vi "Chart_Data_Packer.vi"(0 "DataCluster":T2={"Core"={"Current VI Reference"=refnum, "Close Panel on Exit?"=FALSE, "Exit"=FALSE, "Initialized?"=FALSE}, "Connections"={"cDAQ"={"Task"="", "Connected"=FALSE, "Active"=FALSE, "ID"=""}, "Camera"={"Session"="", "Connected"=FALSE, "Active"=FALSE, "Placeholder"=refnum}, "PSU"={"Port"="", "Connected"=FALSE, "Active"=FALSE}, "Arduino"={"Port"="", "Connected"=FALSE, "Active"=FALSE}}, "Data Acquisition"={"Setup"={"Label"="", "Operator"="", "Notes"="", "TempGrad"=1.0, "TargetTemp"=1.0, "Sample Volume"=1.0}, "Camera"={"Image"=refnum, "Save Image"=refnum, "Image Frequency"=20, "Rectangle"={"Left"=0, "Top"=0, "Right"=0, "Bottom"=0, "Rotation"=0.0}, "Calibration"={"Top Left"={"X"=0.0, "Y"=0.0}, "Top Right"={"X"=0.0, "Y"=0.0}, "Bottom Left"={"X"=0.0, "Y"=0.0}, "Bottom Right"={"X"=0.0, "Y"=0.0}, "Fixpoint"={"X"=0.0, "Y"=0.0}, "Scan Area"=0.0, "Fixpoint Area"=0.0, "Well Pixels"=[], "Valid"=FALSE}, "FocusPos"=0, "Display Mapping"=10, "Camera Mode"=10}, "Thermistor"={"Sample Size"=1, "Calibration"={"B0.100"=[], "R25"=[], "c"=[], "State"=[], "V_S"=5.0, "R_S"=100.0}, "Timing Mode"=14713}, "Partition"={"Data"=[], "Cell Label"="", "Cell Color"=0, "Height"=10, "Width"=16, "Grid"=[]}, "Queue"={"Size"=1, "Queue"=refnum}, "Sample Rate"=1, "Active"=FALSE, "Ready"=FALSE, "Graph Mode"=0, "Gradient Buffer"=2}, "Control"={"Sample Rate"=1, "PID gains"={"proportional gain (Kc)"=1.0, "integral time (Ti, min)"=0.01, "derivative time (Td, min)"=0.0}}, "Manual Temp Control"={"TargetTemp"=1.0, "Mode"=0, "Active"=FALSE}} {"Manual Temp Control"."Mode" items=["Cool", "Heat"]; "Manual Temp Control"."TargetTemp" min=-40.0 max=40.0 step=0.5 format="%#_g °C"; "Control"."PID gains"."derivative time (Td, min)" format="%.3f"; "Control"."PID gains"."integral time (Ti, min)" format="%.3f"; "Control"."PID gains"."proportional gain (Kc)" format="%.3f"; "Control"."Sample Rate" min=1 max=20 step=1 format="%.0f Samples/sec"; "Data Acquisition"."Gradient Buffer" min=2 max=30 step=1; "Data Acquisition"."Graph Mode" items=["Thermistor Temperature", "Camera Temperature"]; "Data Acquisition"."Thermistor"."Timing Mode" items=["Automatic"=16097, "High Resolution"=10195, "High Speed"=14712, "Best 50 Hz Rejection"=14713, "Best 60 Hz Rejection"=14714, "Custom"=10137]; "Data Acquisition"."Thermistor"."Calibration"."R_S" min=0.1 max=1000.0 format="%#_g kOhm"; "Data Acquisition"."Thermistor"."Calibration"."V_S" min=5.0 max=48.0 format="%#_g V"; "Data Acquisition"."Thermistor"."Calibration"."R25" min=0.1 max=1000.0 format="%#_g kOhm"; "Data Acquisition"."Thermistor"."Calibration"."B0.100" min=100.0 max=10000.0 format="%#_g K"; "Data Acquisition"."Thermistor"."Sample Size" min=1 max=200; "Data Acquisition"."Sample Rate" min=20 max=240 format="%.0f samples/min"; "Data Acquisition"."Queue"."Size" min=1 max=200; "Data Acquisition"."Camera"."Camera Mode" items=["Temperature Linear", "Signal Linear"]; "Data Acquisition"."Camera"."Display Mapping" items=["Default"=10, "Most Significant Bits"=11, "Full Dynamic"=12, "Downshift"=13, "Given Range"=14, "90% Dynamic"=15, "Given Percent Range"=16]; "Data Acquisition"."Camera"."Calibration"."Fixpoint"."Y" format="%.2f"; "Data Acquisition"."Camera"."Calibration"."Fixpoint"."X" format="%.2f"; "Data Acquisition"."Camera"."Calibration"."Top Left"."Y" format="%.2f"; "Data Acquisition"."Camera"."Calibration"."Top Left"."X" format="%.2f"; "Data Acquisition"."Camera"."Calibration"."Top Right"."Y" format="%.2f"; "Data Acquisition"."Camera"."Calibration"."Top Right"."X" format="%.2f"; "Data Acquisition"."Camera"."Calibration"."Bottom Left"."Y" format="%.2f"; "Data Acquisition"."Camera"."Calibration"."Bottom Left"."X" format="%.2f"; "Data Acquisition"."Camera"."Calibration"."Bottom Right"."Y" format="%.2f"; "Data Acquisition"."Camera"."Calibration"."Bottom Right"."X" format="%.2f"; "Data Acquisition"."Camera"."Rectangle"."Rotation" min=-90.0 max=90.0 step=1.0 format="%.2f"; "Data Acquisition"."Camera"."Rectangle"."Left" scale=0.0..1024.0; "Data Acquisition"."Camera"."Rectangle"."Right" scale=0.0..1024.0; "Data Acquisition"."Camera"."Image Frequency" min=1 max=60 step=1; "Data Acquisition"."Setup"."Sample Volume" min=0.0 max=500.0 format="%#_g µL"; "Data Acquisition"."Setup"."TargetTemp" min=-40.0 max=40.0 step=0.5 format="%#_g °C"; "Data Acquisition"."Setup"."TempGrad" min=-100.0 max=100.0 step=0.1 format="%#_g °C/min"}, 5 "Mean Temperature":dbl format="%0.2f", 7 "Temperatures":dbl[](array[numeric]), 9 "Temp Gradient":dbl, 11 "Reading Cluster in":T1) -> (4 "Chart Data":waveform(dbl)[](array[waveform]), 6 "Gradients":waveform(dbl)[](array[waveform]), 8 "Temps":waveform(dbl)[](array[waveform]), 15 "Reading Cluster":T1)   [LabVIEW 2024]
uses:
  DataCluster.ctl
  <vilib>/userDefined/High Color/IMAQdx.ctl
  <vilib>/vision/Image Controls.llb/IMAQ Image.ctl
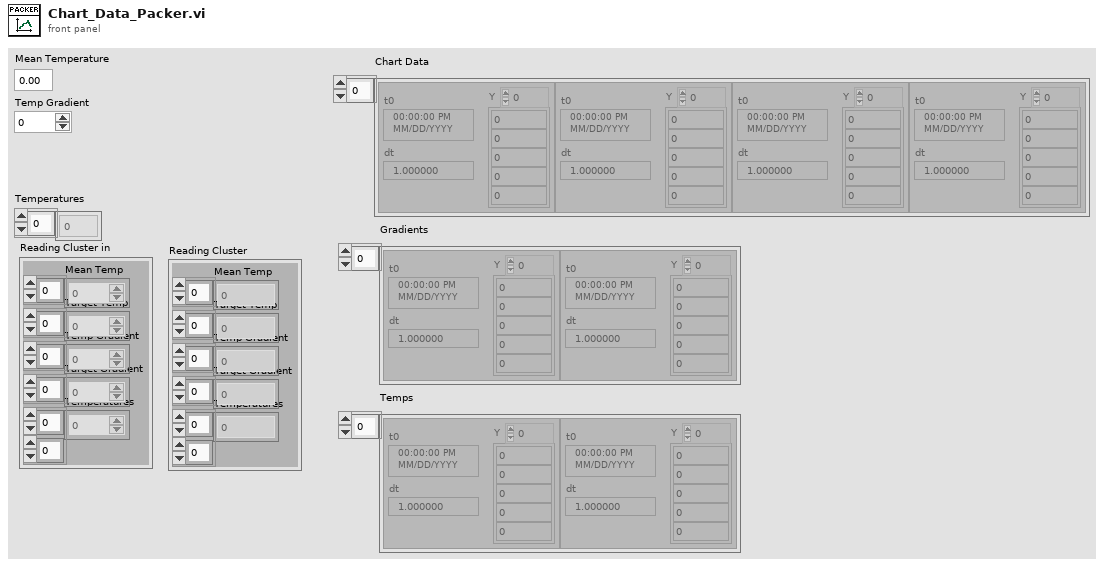
[diagram p1: front panel]
types:
  T1 = cluster{"Mean Temp":dbl[], "Target Temp":dbl[], "Temp Gradient":dbl[], "Target Gradient":dbl[], "Temperatures":dbl[][]}
  T2 = typedef "DataCluster.ctl" = cluster{"Core":cluster{"Current VI Reference":refnum<vi>, "Close Panel on Exit?":bool, "Exit":bool, "Initialized?":bool}, "Connections":cluster{"cDAQ":cluster{"Task":refnum<k21>, "Connected":bool, "Active":bool, "ID":string}, "Camera":cluster{"Session":T3, "Connected":bool, "Active":bool, "Placeholder":T4}, "PSU":cluster{"Port":refnum<visa-resource-name>, "Connected":bool, "Active":bool}, "Arduino":cluster{"Port":refnum<visa-resource-name>, "Connected":bool, "Active":bool}}, "Data Acquisition":cluster{"Setup":cluster{"Label":string, "Operator":string, "Notes":string, "TempGrad":dbl, "TargetTemp":dbl, "Sample Volume":dbl}, "Camera":cluster{"Image":T4, "Save Image":T4, "Image Frequency":i32, "Rectangle":T5, "Calibration":cluster{"Top Left":T6, "Top Right":T6, "Bottom Left":T6, "Bottom Right":T6, "Fixpoint":T6, "Scan Area":dbl, "Fixpoint Area":dbl, "Well Pixels":cluster{"X":i32, "Y":i32}[][], "Valid":bool}, "FocusPos":u32, "Display Mapping":u32, "Camera Mode":u32}, "Thermistor":cluster{"Sample Size":i32, "Calibration":cluster{"B0.100":dbl[], "R25":dbl[], "c":dbl[][], "State":bool[], "V_S":dbl, "R_S":dbl}, "Timing Mode":i32}, "Partition":cluster{"Data":string[][], "Cell Label":string, "Cell Color":u32, "Height":i32, "Width":i32, "Grid":string[][]}, "Queue":cluster{"Size":i32, "Queue":refnum<queue>}, "Sample Rate":i32, "Active":bool, "Ready":bool, "Graph Mode":u16, "Gradient Buffer":i32}, "Control":cluster{"Sample Rate":i32, "PID gains":cluster{"proportional gain (Kc)":dbl, "integral time (Ti, min)":dbl, "derivative time (Td, min)":dbl}}, "Manual Temp Control":cluster{"TargetTemp":dbl, "Mode":u16, "Active":bool}}
  T3 = typedef "IMAQdx.ctl" = refnum<k21>
  T4 = typedef "IMAQ Image.ctl" = refnum<image>
  T5 = typedef "IMAQ Rectangle" = cluster{"Left":i32, "Top":i32, "Right":i32, "Bottom":i32, "Rotation":dbl}
  T6 = typedef "IMAQ Point" = cluster{"X":sgl, "Y":sgl}
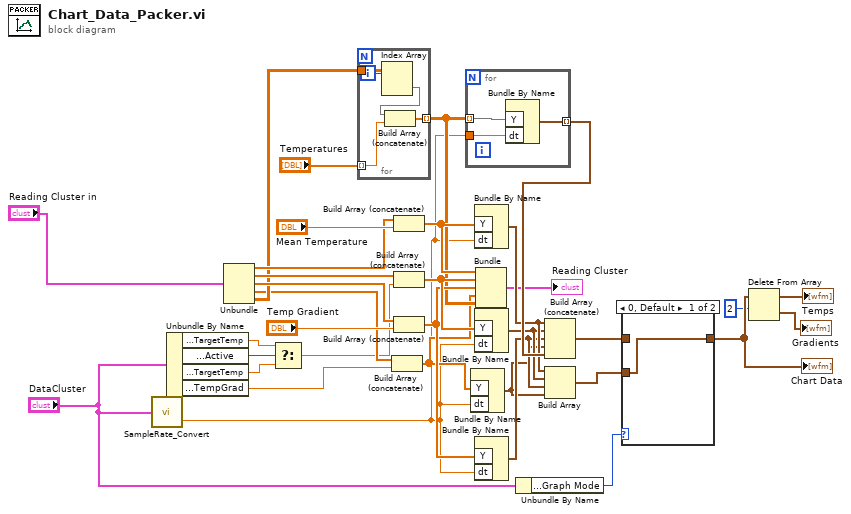
[diagram p0: block diagram]
diagram:
  n1 = call "SampleRate_Convert.vi"("DataCluster"="DataCluster") -> ("Sample dt (s)"=w11:dbl)  [unwired: 1 out]
  n2 = Unbundle By Name("DataCluster") -> ("Manual Temp Control.TargetTemp"=w3:dbl, "Manual Temp Control.Active"=w4:bool, "Data Acquisition.Setup.TargetTemp"=w5:dbl, "Data Acquisition.Setup.TempGrad"=w16:dbl)
  n3 = Unbundle("Reading Cluster in") -> ("Mean Temp"=w27:dbl[], "Target Temp"=w28:dbl[], "Temp Gradient"=w29:dbl[], "Target Gradient"=w13:dbl[], "Temperatures"=w14:dbl[][])
  n4 = Select(t=w3, s=w4, f=w5) -> (s? t:f=w2:dbl)
  n5 = for {
    tunnel: "Temperatures" -> [w39] mode=indexing
    tunnel: [w38] -> w25 mode=indexing
    tunnel: w14 -> [w36]
    i -> [w37]
    n6 = Index Array(array=w36, index (row)=w37) -> (element=w35:dbl[])  [unwired: 1 in]
    n7 = Build Array (concatenate)(w35, w39) -> (w38:dbl[])
  }
  n8 = Build Array (concatenate)(w13, w16) -> (w12:dbl[])
  n9 = Build Array (concatenate)(w27, "Mean Temperature") -> (w32:dbl[])
  n10 = Build Array (concatenate)(w28, w2) -> (w33:dbl[])
  n11 = Build Array (concatenate)(w29, "Temp Gradient") -> (w30:dbl[])
  n12 = for {
    tunnel: w25 -> [w42] mode=indexing
    tunnel: w11 -> [w41]
    tunnel: [w40] -> w24 mode=indexing
    n13 = Bundle By Name("Y"=w42, "dt"=w41) -> (w40:waveform(dbl))  [unwired: 1 in]
  }
  n14 = Bundle By Name("Y"=w12, "dt"=w11) -> (w10:waveform(dbl))  [unwired: 1 in]
  n15 = Bundle By Name("Y"=w32, "dt"=w11) -> (w21:waveform(dbl))  [unwired: 1 in]
  n16 = Bundle By Name("Y"=w33, "dt"=w11) -> (w20:waveform(dbl))  [unwired: 1 in]
  n17 = Bundle By Name("Y"=w30, "dt"=w11) -> (w19:waveform(dbl))  [unwired: 1 in]
  n18 = Bundle(w32, w33, w30, w12, w25) -> (→"Reading Cluster":cluster{dbl[], dbl[], dbl[], dbl[], dbl[][]})  [unwired: 1 in]
  n19 = Unbundle By Name("DataCluster") -> ("Data Acquisition.Graph Mode"=w22:u16)
  n20 = Build Array (concatenate)(w21, w20, w19, w10, w24) -> (w18:waveform(dbl)[])
  n21 = Build Array(w21, w20, w19, w10) -> (w17:waveform(dbl)[])
  n22 = case shown="0, Default" w22 {
    tunnel: w18 -> [_ w44]
    tunnel: w17 -> [w43 _]
    tunnel: [w43 w44] -> w9
    frame 0, Default {
    }
    frame 1 {
    }
  }
  "Chart Data" <- w9
  n23 = Delete From Array(array=w9, length=2) -> (deleted portion=→"Gradients":waveform(dbl)[], array with subset deleted=→"Temps":waveform(dbl)[])  [unwired: 1 in]
